vi "Processing Step.vi"(8 "error in (no error)":errorcluster, 11 "TestCSRFController in":refnum<class "TestCSRFController.lvclass">) -> (0 "error out":errorcluster, 2 "Array":T1[](array[typedef]), 3 "TestCSRFController out":refnum<class "TestCSRFController.lvclass">)   [LabVIEW 2020, in "TestCSRFController.lvclass"]
uses:
  TestCSRFController.lvclass
  HTTP Server/Processing Step.ctl
  HTTP Server/HTTP Server.lvlib
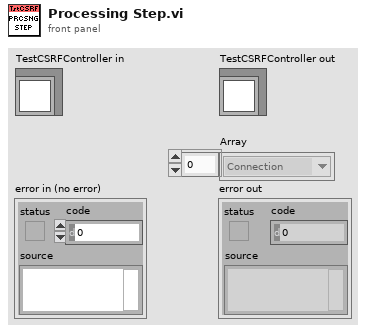
[diagram p1: front panel]
types:
  T1 = typedef "HTTP Server.lvlib/Processing Step.ctl" = enum16{"Connection", "Request", "Routing", "Controller Init", "Controller", "Response", "Complete", "Exception"}
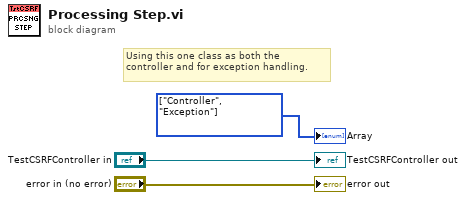
[diagram p0: block diagram]
diagram:
  w1 = T1[] [enum."Controller", enum."Exception"] items=["Connection", "Request", "Routing", "Controller Init", "Controller", "Response", "Complete", "Exception"] ("Array")
  # "Using this one class as both the controller and for exception handling."
  "error out" <- "error in (no error)"
  "TestCSRFController out" <- "TestCSRFController in"
  "Array" <- w1
